vi "X_LMS_Notch15.vi"(4 "eta":dbl=-500.0 format="%#_13g", 5 "ek":dbl format="%#_13g", 6 "q_input":dbl[](array[numeric])=[4332.68720809435, -762.824007058915, 3079.39627759621, -548.742069565578, 583.662600399268, -139.519105490218, 531.489726955241, 465.655333713069, 1073.86410215099, 808.069244251544, 1769.88829799787, 469.778970291169, -433.911680836792, 3754.02296145848, -7477.2140366405], 7 "Bound":dbl=100000.0 format="%.4f", 9 "phik":dbl[](array[numeric])=[915.3955183085, 84.33546198759, -358.8100229269, -15.56872770464, 872.6860692726]) -> (0 "q_out":dbl[](array[numeric]))   [LabVIEW 2015]
panel:
  in  "Notch4352":T1={"w0"=100000.0, "constrints"=[{"beta"=[-19381.69245689673, -19381.69435374671, -19381.696056779747, -19381.697565995823, -19381.698881394925, -19381.700002977042, -19381.70093074215, -19381.701664690256, -19381.70220482134, -19381.70255113541, -19381.702703632447, -19381.702662312462, -19381.702427175453, -19381.70199822141, -19381.701375450357], "gamma"=-268840077.40019166, "OmegaChain"=[0.99999902000016, 0.999999155000119, 0.9999992800000864, 0.999999395000061, 0.9999995000000417, 0.9999995950000273, 0.999999680000017, 0.99999975500001, 0.9999998200000054, 0.9999998750000026, 0.999999920000001, 0.9999999550000004, 0.9999999800000001, 0.999999995, 1.0, 0.999999995, 0.9999999800000001, 0.9999999550000004, 0.999999920000001, 0.9999998750000026, 0.9999998200000054, 0.99999975500001, 0.999999680000017, 0.9999995950000273, 0.9999995000000417, 0.999999395000061, 0.9999992800000864, 0.999999155000119, 0.99999902000016], "weight"=5e-07}, {"beta"=[-19385.216000946515, -19385.405735674605, -19385.576084998575, -19385.727048748067, -19385.858626772133, -19385.97081893919, -19386.063625137038, -19386.137045272877, -19386.19107927329, -19386.22572708424, -19386.24098867107, -19386.236864018534, -19386.213353130748, -19386.17045603122, -19386.10817276286], "gamma"=-268841192.1136133, "OmegaChain"=[0.9999020016006562, 0.9999155011900349, 0.9999280008639958, 0.9999395006100392, 0.9999500004166653, 0.9999595002733742, 0.9999680001706663, 0.9999755001000415, 0.999982000054, 0.9999875000260416, 0.9999920000106667, 0.999995500003375, 0.9999980000006666, 0.9999995000000417, 1.0, 0.9999995000000417, 0.9999980000006666, 0.999995500003375, 0.9999920000106667, 0.9999875000260416, 0.999982000054, 0.9999755001000415, 0.9999680001706663, 0.9999595002733742, 0.9999500004166653, 0.9999395006100392, 0.9999280008639958, 0.9999155011900349, 0.9999020016006562], "weight"=5e-07}, {"beta"=[-19735.867778631145, -19755.33494552827, -19772.826595393555, -19788.34097907661, -19801.87654515198, -19813.431940074355, -19823.00600831385, -19830.597792471628, -19836.206533375615, -19839.831670156367, -19841.47284030325, -19841.129879700606, -19838.80282264421, -19834.491901837835, -19828.197548369964], "gamma"=-269025159.2772959, "OmegaChain"=[0.9902159962126371, 0.9915618937147881, 0.9928086358538663, 0.9939560979566968, 0.9950041652780257, 0.9959527330119943, 0.9968017063026194, 0.9975510002532796, 0.9982005399352042, 0.9987502603949663, 0.9992001066609779, 0.9995500337489875, 0.9998000066665778, 0.9999500004166653, 1.0, 0.9999500004166653, 0.9998000066665778, 0.9995500337489875, 0.9992001066609779, 0.9987502603949663, 0.9982005399352042, 0.9975510002532796, 0.9968017063026194, 0.9959527330119943, 0.9950041652780257, 0.9939560979566968, 0.9928086358538663, 0.9915618937147881, 0.9902159962126371], "weight"=5e-07}, {"beta"=[-125979.56827796053, -137840.02384521344, -148323.227458059, -157324.43441128405, -164753.70762041546, -170536.81624333866, -174615.9773703351, -176950.43337181513, -177516.85913508057, -176309.59512114027, -173340.70391295323, -168639.8496900866, -162254.0018340394, -154246.96562570872, -144698.74472411387], "gamma"=-800788288.0111153, "OmegaChain"=[0.16996714290024081, 0.26749882862458735, 0.3623577544766736, 0.4535961214255773, 0.5403023058681398, 0.6216099682706644, 0.6967067093471654, 0.7648421872844884, 0.8253356149096783, 0.8775825618903728, 0.9210609940028851, 0.955336489125606, 0.9800665778412416, 0.9950041652780257, 1.0, 0.9950041652780257, 0.9800665778412416, 0.955336489125606, 0.9210609940028851, 0.8775825618903728, 0.8253356149096783, 0.7648421872844884, 0.6967067093471654, 0.6216099682706644, 0.5403023058681398, 0.4535961214255773, 0.3623577544766736, 0.26749882862458735, 0.16996714290024081], "weight"=5e-07}, {"beta"=[6171.821347036184, 4645.94730687319, 2386.580342071111, -249.5751826016643, -2846.3282736021943, -4993.7087152834365, -6352.692352517477, -6708.725550325106, -6005.5984952325125, -4354.319488877073, -2015.589178029993, 641.3583452415528, 3197.049487990446, 5247.996813328242, 6470.400834825722], "gamma"=-106065386.2489967, "OmegaChain"=[0.7755658785102502, 0.4685166713003771, 0.0874989834394464, -0.30733286997841935, -0.6536436208636119, -0.896758416334147, -0.9982947757947531, -0.9422223406686583, -0.7373937155412454, -0.4161468365471424, -0.029199522301288815, 0.3623577544766736, 0.6967067093471654, 0.9210609940028851, 1.0, 0.9210609940028851, 0.6967067093471654, 0.3623577544766736, -0.029199522301288815, -0.4161468365471424, -0.7373937155412454, -0.9422223406686583, -0.9982947757947531, -0.896758416334147, -0.6536436208636119, -0.30733286997841935, 0.0874989834394464, 0.4685166713003771, 0.7755658785102502], "weight"=5e-07}, {"beta"=[-1035.2700299602095, -630.7064176273165, -71.7238776039502, 504.8191691145451, 957.7648770497714, 1176.2163398653695, 1106.689020702965, 766.205632143542, 238.12838247975833, -348.25100023274865, -849.3663924100385, -1142.5272690368206, -1155.9576231718522, -886.3692357228977, -399.76674616117367], "gamma"=-45864717.01307516, "OmegaChain"=[0.7539022543433046, 0.9765876257280235, 0.9601702866503661, 0.70866977429126, 0.28366218546322625, -0.2107957994307797, -0.6536436208636119, -0.9364566872907963, -0.9899924966004454, -0.8011436155469337, -0.4161468365471424, 0.0707372016677029, 0.5403023058681398, 0.8775825618903728, 1.0, 0.8775825618903728, 0.5403023058681398, 0.0707372016677029, -0.4161468365471424, -0.8011436155469337, -0.9899924966004454, -0.9364566872907963, -0.6536436208636119, -0.2107957994307797, 0.28366218546322625, 0.70866977429126, 0.9601702866503661, 0.9765876257280235, 0.7539022543433046], "weight"=5e-07}, {"beta"=[-3079.156564752011, -1428.3477809910216, 721.4239764938134, 2619.1815834912336, 3601.9837090478723, 3326.509295312105, 1888.989480450481, -208.40870650108369, -2233.0037363156825, -3477.546317114347, -3507.281919709228, -2311.8230426152772, -308.7778651692609, 1802.1323041753387, 3283.50581199956], "gamma"=-26192083.44782192, "OmegaChain"=[-0.5192886541166856, 0.05395542056264975, 0.6083513145322546, 0.9502325919585293, 0.9601702866503661, 0.6346928759426347, 0.0874989834394464, -0.4902608213406994, -0.896758416334147, -0.9899924966004454, -0.7373937155412454, -0.2272020946930871, 0.3623577544766736, 0.8253356149096783, 1.0, 0.8253356149096783, 0.3623577544766736, -0.2272020946930871, -0.7373937155412454, -0.9899924966004454, -0.896758416334147, -0.4902608213406994, 0.0874989834394464, 0.6346928759426347, 0.9601702866503661, 0.9502325919585293, 0.6083513145322546, 0.05395542056264975, -0.5192886541166856], "weight"=5e-07}, {"beta"=[-3573.2183742405814, -877.3708025653453, 2231.11796685333, 4290.2770942809875, 4331.651866839491, 2335.7830824959196, -758.6409831629235, -3496.264340347889, -4589.539947629954, -3524.2832040017724, -801.5010010874465, 2298.2396464369126, 4317.082277256923, 4305.533656811656, 2269.0252817486935], "gamma"=-16189144.802904319, "OmegaChain"=[-0.9304262721047533, -0.9477216021311119, -0.5192886541166856, 0.15337386203786435, 0.7539022543433046, 0.9998586363834151, 0.7755658785102502, 0.18651236942257576, -0.4902608213406994, -0.9364566872907963, -0.9422223406686583, -0.5048461045998576, 0.16996714290024081, 0.7648421872844884, 1.0, 0.7648421872844884, 0.16996714290024081, -0.5048461045998576, -0.9422223406686583, -0.9364566872907963, -0.4902608213406994, 0.18651236942257576, 0.7755658785102502, 0.9998586363834151, 0.7539022543433046, 0.15337386203786435, -0.5192886541166856, -0.9477216021311119, -0.9304262721047533], "weight"=5e-07}, {"beta"=[-3343.4470711032995, 122.18872893498246, 3513.7064856145075, 4773.857037473571, 3138.2499693295317, -400.9774189927299, -3696.9772855474203, -4750.440339297189, -2922.350027936131, 678.3985962492302, 3867.6397351732057, 4710.822509416504, 2696.483562535053, -953.5061300914715, -4025.1117990118105], "gamma"=-9656153.96067803, "OmegaChain"=[0.20300486381875213, -0.5609842574272288, -0.984687855794127, -0.811093014061656, -0.14550003380861354, 0.6083513145322546, 0.9931849187581926, 0.7755658785102502, 0.0874989834394464, -0.6536436208636119, -0.9982947757947531, -0.7373937155412454, -0.029199522301288815, 0.6967067093471654, 1.0, 0.6967067093471654, -0.029199522301288815, -0.7373937155412454, -0.9982947757947531, -0.6536436208636119, 0.0874989834394464, 0.7755658785102502, 0.9931849187581926, 0.6083513145322546, -0.14550003380861354, -0.811093014061656, -0.984687855794127, -0.5609842574272288, 0.20300486381875213], "weight"=5e-07}, {"beta"=[-2849.5230367762247, 1023.2933835990091, 4121.701772197345, 4100.888432074458, 976.6044840893321, -2886.7542673389416, -4565.474941140862, -2789.1351992672285, 1097.9664557026724, 4154.14898665041, 4066.554383864078, 901.4724963989494, -2945.825804097223, -4563.781865630508, -2727.958797280408], "gamma"=-4882673.16129464, "OmegaChain"=[0.9994345855010047, 0.6475963386538773, -0.1943299064553348, -0.8891911526253609, -0.9111302618846769, -0.2435441537357911, 0.6083513145322546, 0.9998586363834151, 0.6346928759426347, -0.2107957994307797, -0.896758416334147, -0.9040721420170612, -0.2272020946930871, 0.6216099682706644, 1.0, 0.6216099682706644, -0.2272020946930871, -0.9040721420170612, -0.896758416334147, -0.2107957994307797, 0.6346928759426347, 0.9998586363834151, 0.6083513145322546, -0.2435441537357911, -0.9111302618846769, -0.8891911526253609, -0.1943299064553348, 0.6475963386538773, 0.9994345855010047], "weight"=5e-07}, {"beta"=[-2367.916072856672, 1600.5334310208036, 4097.459879655843, 2827.20061133968, -1042.373860738555, -3953.594612407114, -3229.89871036428, 463.35117054641114, 3730.598122110136, 3567.950364740505, 124.94549647459453, -3432.93368503438, -3834.589468307564, -710.7413785341431, 3066.55905691177], "gamma"=-1138287.5404370662, "OmegaChain"=[0.1367372182078336, 0.9074467814501962, 0.8438539587324921, 0.004425697988050785, -0.8390715290764524, -0.9111302618846769, -0.14550003380861354, 0.7539022543433046, 0.9601702866503661, 0.28366218546322625, -0.6536436208636119, -0.9899924966004454, -0.4161468365471424, 0.5403023058681398, 1.0, 0.5403023058681398, -0.4161468365471424, -0.9899924966004454, -0.6536436208636119, 0.28366218546322625, 0.9601702866503661, 0.7539022543433046, -0.14550003380861354, -0.9111302618846769, -0.8390715290764524, 0.004425697988050785, 0.8438539587324921, 0.9074467814501962, 0.1367372182078336], "weight"=5e-07}, {"beta"=[-2347.0577358436576, 2000.4104815875623, 3417.272657029697, -172.1776158950111, -3509.387278164276, -1705.3363563029345, 2597.036322720362, 3094.7447047493406, -941.3551558951775, -3598.367507792691, -983.7630306954654, 3072.05659108227, 2627.3061098613666, -1666.4539774299908, -3518.855083699983], "gamma"=-6339513.789849784, "OmegaChain"=[0.7963524702919231, -0.36976826386317313, -0.9941776251838151, -0.16211443649971827, 0.9074467814501962, 0.6475963386538773, -0.5609842574272288, -0.9477216021311119, 0.05395542056264975, 0.9765876257280235, 0.4685166713003771, -0.7259323042001402, -0.8568887533689473, 0.26749882862458735, 1.0, 0.26749882862458735, -0.8568887533689473, -0.7259323042001402, 0.4685166713003771, 0.9765876257280235, 0.05395542056264975, -0.9477216021311119, -0.5609842574272288, 0.6475963386538773, 0.9074467814501962, -0.16211443649971827, -0.9941776251838151, -0.36976826386317313, 0.7963524702919231], "weight"=5e-07}, {"beta"=[-2637.239994230651, 2605.8278869119135, 3005.897939726276, -2180.570269402013, -3314.3928175208507, 1711.6685231240967, 3556.550100537828, -1208.5077197180296, -3727.5230091111675, 681.1586260850307, 3823.889519313312, -140.1761379196681, -3843.7208547873597, -403.61197659922965, 3786.6200912189593], "gamma"=-23969209.399015553, "OmegaChain"=[-0.5477292602242684, 0.7958149698139441, 0.6603167082440802, -0.7023970575027135, -0.7596879128588213, 0.594920663309892, 0.8438539587324921, -0.47553692799599256, -0.9111302618846769, 0.3466353178350258, 0.9601702866503661, -0.2107957994307797, -0.9899924966004454, 0.0707372016677029, 1.0, 0.0707372016677029, -0.9899924966004454, -0.2107957994307797, 0.9601702866503661, 0.3466353178350258, -0.9111302618846769, -0.47553692799599256, 0.8438539587324921, 0.594920663309892, -0.7596879128588213, -0.7023970575027135, 0.6603167082440802, 0.7958149698139441, -0.5477292602242684], "weight"=5e-07}, {"beta"=[-2403.694272801173, 3467.7735291100403, 827.9234533310928, -3843.9854147947585, 918.799623090996, 3426.4790168557724, -2475.8060431940794, -2301.462378720777, 3521.600189799468, 701.2324991327548, -3840.2431751391273, 1043.7900879121328, 3365.9405863520888, -2573.2875915754826, -2196.6279242447395], "gamma"=-57938868.307501644, "OmegaChain"=[0.9977389813911304, -0.16123796432418536, -0.9244717749141217, 0.5813218118144357, 0.6603167082440802, -0.8813724903622346, -0.25981735621375585, 0.9994345855010047, -0.1943299064553348, -0.9111302618846769, 0.6083513145322546, 0.6346928759426347, -0.896758416334147, -0.2272020946930871, 1.0, -0.2272020946930871, -0.896758416334147, 0.6346928759426347, 0.6083513145322546, -0.9111302618846769, -0.1943299064553348, 0.9994345855010047, -0.25981735621375585, -0.8813724903622346, 0.6603167082440802, 0.5813218118144357, -0.9244717749141217, -0.16123796432418536, 0.9977389813911304], "weight"=5e-07}, {"beta"=[-1993.6127474644277, 3737.5095573908593, -1117.092810281405, -2807.760279134531, 3453.973926170519, -66.96036664981727, -3398.2432366598027, 2895.296712157215, 988.5061014006678, -3718.024086168088, 2105.981821929192, 1965.228740124847, -3741.6292685181543, 1148.9056271272102, 2785.4023840777563], "gamma"=-94163529.43692411, "OmegaChain"=[-0.9626058663135666, 0.6469193223286404, 0.424179007336997, -0.9999608263946371, 0.40808206181339196, 0.6603167082440802, -0.9576594803233847, 0.1367372182078336, 0.8438539587324921, -0.8390715290764524, -0.14550003380861354, 0.9601702866503661, -0.6536436208636119, -0.4161468365471424, 1.0, -0.4161468365471424, -0.6536436208636119, 0.9601702866503661, -0.14550003380861354, -0.8390715290764524, 0.8438539587324921, 0.1367372182078336, -0.9576594803233847, 0.6603167082440802, 0.40808206181339196, -0.9999608263946371, 0.424179007336997, 0.6469193223286404, -0.9626058663135666], "weight"=5e-07}, {"beta"=[-65.03970753433308, 1907.1497616205274, -2990.7620032939512, 2884.910007498085, -1631.6924645751449, -270.4700064372487, 2065.0631022834245, -3038.354233754572, 2803.253090001517, -1453.2623978792876, -474.7093064506796, 2213.8830580866365, -3072.5672486565813, 2709.2522111130193, -1268.4329750226366], "gamma"=-234322477.12597635, "OmegaChain"=[-0.9036922050915067, 0.4677318402470736, 0.15425144988758405, -0.7148869687796651, 0.9912028118634736, -0.8733046400935156, 0.40808206181339196, 0.2194399632114593, -0.7596879128588213, 0.9977982791785807, -0.8390715290764524, 0.3466353178350258, 0.28366218546322625, -0.8011436155469337, 1.0, -0.8011436155469337, 0.28366218546322625, 0.3466353178350258, -0.8390715290764524, 0.9977982791785807, -0.7596879128588213, 0.2194399632114593, 0.40808206181339196, -0.8733046400935156, 0.9912028118634736, -0.7148869687796651, 0.15425144988758405, 0.4677318402470736, -0.9036922050915067], "weight"=5e-07}, {"beta"=[1828.2563220255067, -1678.7530570345318, 1495.6495381929863, -1282.610583675422, 1043.9001696049866, -784.2960865423157, 508.99431197498603, -223.505012792769, -66.45774074013039, 355.0903421402629, -636.6158079281599, 905.3994039919544, -1156.0614248289405, 1383.5848683877878, -1583.415851398709], "gamma"=-363092997.3888489, "OmegaChain"=[-0.39998531498835127, 0.26664293235993725, -0.12796368962740468, -0.013276747223059479, 0.15425144988758405, -0.2921388087338362, 0.424179007336997, -0.5477292602242684, 0.6603167082440802, -0.7596879128588213, 0.8438539587324921, -0.9111302618846769, 0.9601702866503661, -0.9899924966004454, 1.0, -0.9899924966004454, 0.9601702866503661, -0.9111302618846769, 0.8438539587324921, -0.7596879128588213, 0.6603167082440802, -0.5477292602242684, 0.424179007336997, -0.2921388087338362, 0.15425144988758405, -0.013276747223059479, -0.12796368962740468, 0.26664293235993725, -0.39998531498835127], "weight"=5e-07}], "Nc"=17}
  out "One norm":dbl
  out "deltaJ":dbl[](array[numeric])
  out "fitness":dbl[](array[numeric])
  out ">0":bool[](array[boolean])
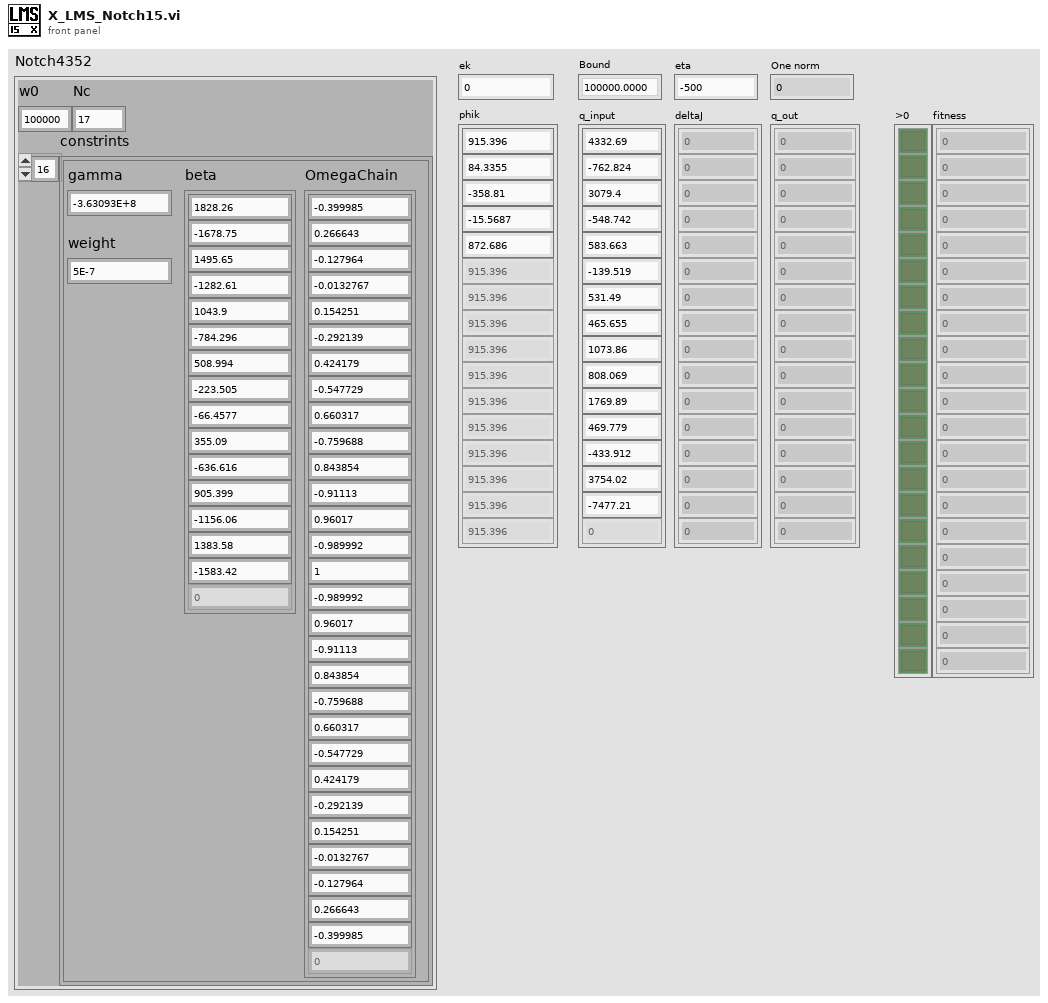
[diagram p1: front panel]
types:
  T1 = cluster{"w0":dbl, "constrints":cluster{"beta":dbl[], "gamma":dbl, "OmegaChain":dbl[], "weight":dbl}[], "Nc":i32}
  T2 = cluster{"beta":dbl[], "gamma":dbl, "OmegaChain":dbl[], "weight":dbl}[]
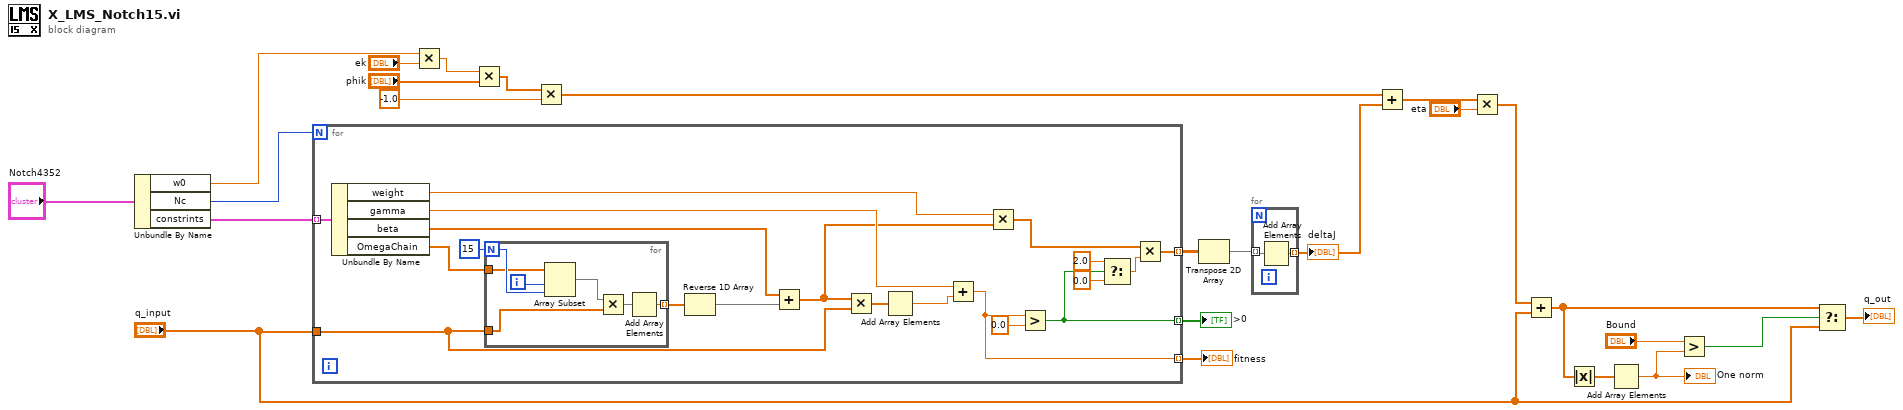
[diagram p0: block diagram]
diagram:
  n1 = Unbundle By Name("Notch4352") -> ("w0"=w3:dbl, "Nc"=w2:i32, "constrints"=w19:T2)
  n2 = for {
    N: w2 -> [_]
    tunnel: "q_input" -> [w39]
    tunnel: w19 -> [w45] mode=indexing
    tunnel: [w32] -> w18 mode=indexing
    tunnel: [w28] -> w15 mode=indexing
    tunnel: [w31] -> w14 mode=indexing
    n3 = Unbundle By Name(w45) -> ("weight"=w33:dbl, "gamma"=w36:dbl, "beta"=w40:dbl[], "OmegaChain"=w42:dbl[])
    n4 = for {
      N: 15 -> [w52]
      tunnel: w39 -> [w48]
      tunnel: w42 -> [w50]
      tunnel: [w46] -> w43 mode=indexing
      i -> [w51]
      n5 = Array Subset(array=w50, index=w51, length=w52) -> (w49:dbl[])
      n6 = Multiply(x=w49, y=w48) -> (x*y=w47:dbl[])
      n7 = Add Array Elements(numeric array=w47) -> (sum=w46:dbl)
    }
    n8 = Reverse 1D Array(array=w43) -> (reversed array=w41:dbl[])
    n9 = Add(x=w40, y=w41) -> (x+y=w30:dbl[])
    n10 = Multiply(x=w30, y=w39) -> (x*y=w38:dbl[])
    n11 = Add Array Elements(numeric array=w38) -> (sum=w37:dbl)
    n12 = Add(x=w36, y=w37) -> (x+y=w31:dbl)
    n13 = Multiply(x=w33, y=w30) -> (x*y=w34:dbl[])
    n14 = Greater?(x=w31, y=0.0) -> (0:w28:bool)
    n15 = Select(t=2.0 ("y"), s=w28, f=0.0) -> (s? t:f=w29:dbl)
    n16 = Multiply(x=w34, y=w29) -> (x*y=w32:dbl[])
  }
  ">0" <- w15
  "fitness" <- w14
  n17 = Multiply(x=w3, y="ek") -> (x*y=w13:dbl)
  n18 = Multiply(x=w13, y="phik") -> (x*y=w12:dbl[])
  n19 = Multiply(x=w12, y=-1.0) -> (x*y=w7:dbl[])
  n20 = Transpose 2D Array(2D array=w18) -> (transposed array=w20:dbl[][])
  n21 = for {
    tunnel: w20 -> [w54] mode=indexing
    tunnel: [w53] -> w8 mode=indexing
    n22 = Add Array Elements(numeric array=w54) -> (sum=w53:dbl)
  }
  "deltaJ" <- w8
  n23 = Add(x=w7, y=w8) -> (x+y=w23:dbl[])
  n24 = Multiply(x=w23, y="eta") -> (x*y=w4:dbl[])
  n25 = Add(x=w4, y="q_input") -> (x+y=w6:dbl[])
  n26 = Absolute Value(x=w6) -> (abs(x)=w17:dbl[])
  n27 = Add Array Elements(numeric array=w17) -> (sum=w16:dbl)
  "One norm" <- w16
  n28 = Greater?(x="Bound", y=w16) -> (0:w21:bool)
  n29 = Select(t=w6, s=w21, f="q_input") -> (s? t:f=→"q_out":dbl[])
